vi "Switch Unflatten Test Parameters.vi"(9 "error in (no error)":errorcluster, 10 "Parameter String":string) -> (1 "error out":errorcluster, 2 "Switch Test Parameters":T2, 5 "Test Version":string)   [LabVIEW 2011]
uses:
  TypeDefs/Switch Test Parameters.ctl
  TypeDefs/Switch Stimulus Parameters.ctl
  TypeDefs/Switch Type.ctl
  TypeDefs/Switch Instrument Info.ctl
  Test Return Parameter.ctl
  TypeDefs/Switch Test Parameters v5.3-5.4.ctl
  TypeDefs/Switch Test Parameters v5.5.ctl
panel:
  in  "Return Parameter":T1
  out "Parameter Variant":variant
  in  "Required Instruments":string[](array[string])=["SWI_PFE"]
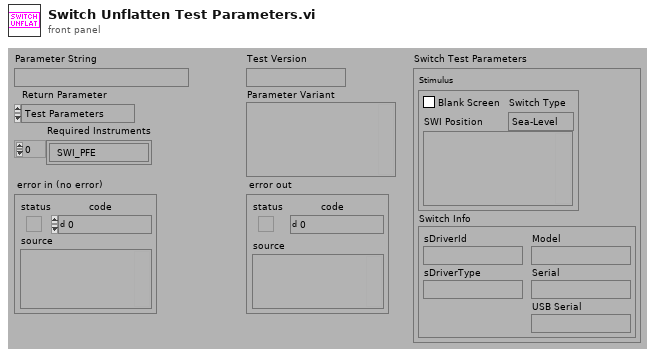
[diagram p1: front panel]
types:
  T1 = typedef "Test Return Parameter.ctl" = enum16{"Test Parameters", "Required Instruments", "Datasheets", "QuickMode"}
  T2 = typedef "Switch Test Parameters.ctl" = cluster{"Stimulus":T3, "Switch Info":T5}
  T3 = typedef "Switch Stimulus Parameters.ctl" = cluster{"Blank Screen":bool, "SWI Position":variant, "Switch Type":T4}
  T4 = typedef "Switch Type.ctl" = enum16{"Sea-Level", "Simulator", "SI-0206-SW", "SI-0309-SW", "SI-0310-SW", "Front End"}
  T5 = typedef "Switch Instrument Info.ctl" = cluster{"sDriverId":string, "sDriverType":string, "Model":string, "Serial":string, "USB Serial":string}
  T6 = typedef "Switch Test Parameters v5.3-5.4.ctl" = cluster{"Stimulus":cluster{"Blank Screen":bool, "SWI Position":variant}, "Switch Info":cluster{"sDriverId":string, "Model":string, "Serial":string}}
  T7 = typedef "Switch Test Parameters v5.5.ctl" = cluster{"Stimulus":cluster{"Blank Screen":bool, "SWI Position":variant, "Switch Type":enum16{"Sea-Level", "Simulator", "SI-0206-SW", "SI-0310-SW", "Front End"}}, "Switch Info":cluster{"sDriverId":string, "sDriverType":string, "Model":string, "Serial":string, "USB Serial":string}}
  T8 = enum16{"Sea-Level", "Simulator", "SI-0206-SW", "SI-0310-SW", "Front End"}
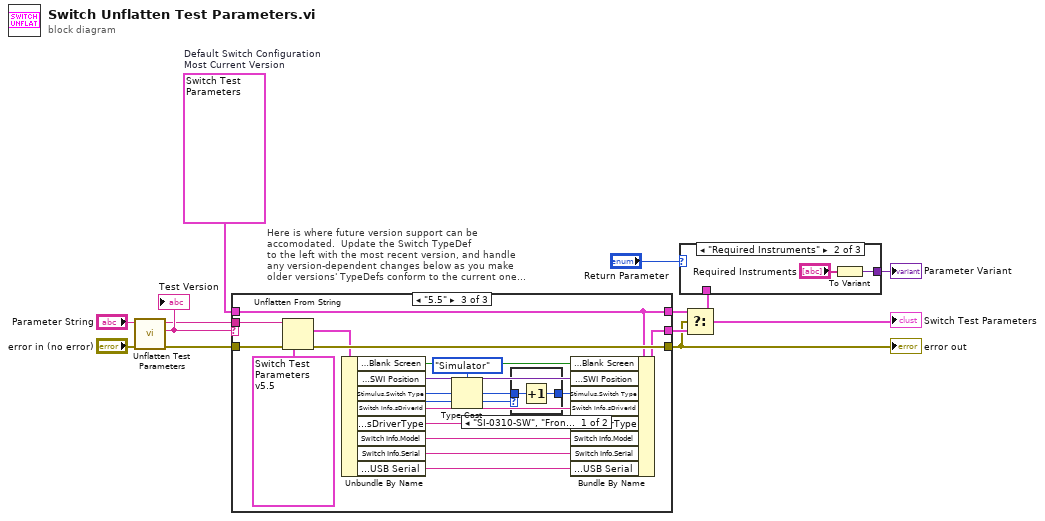
[diagram p0: block diagram]
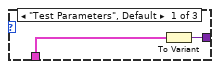
[diagram p2: hidden frame]
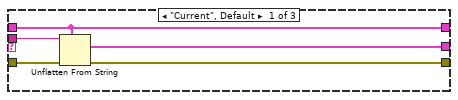
[diagram p4: hidden frame]
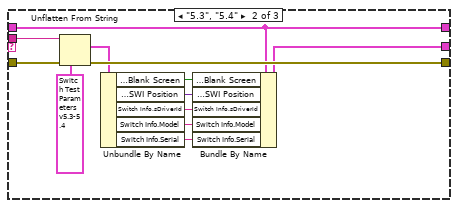
[diagram p5: hidden frame]
diagram:
  w2 = T2 {"Stimulus"={"Blank Screen"=FALSE, "SWI Position"=variant, "Switch Type"=enum."Simulator"}, "Switch Info"={"sDriverId"="", "sDriverType"="", "Model"="", "Serial"="", "USB Serial"=""}}  # Default Switch Configuration Most Current Version
  # "Here is where future version support can be\naccomodated.  Update the Switch TypeDef\nto the left with the most recent version, and handle\nany version-dependent changes below as you make\nolder versions' TypeDefs conform to the current one..."
  n1 = call "Unflatten Test Parameters.vi"("error in (no error)"="error in (no error)", "Flattened Test Parameters with Version (\"\")"="Parameter String") -> ("error out"=w3:errorcluster, "Test Version"=w11:string, "Flat Test Parameters"=w10:string)  [unwired: 3 out]
  "Test Version" <- w11
  n2 = case shown="\"5.5\"" w11 {
    tunnel: [w16 w23 w42] -> w9
    tunnel: w10 -> [w17 w29 w47]
    tunnel: [w14 w27 w45] -> w4
    tunnel: w3 -> [w15 w28 w46]
    tunnel: w2 -> [w13 w24 w43]
    tunnel: [w13 w24 w43] -> w1
    frame "Current", Default {
      n3 = Unflatten From String(type=w13, binary string=w17, error in (no error)=w15) -> (value=w16:T2, error out=w14:errorcluster)  [unwired: 3 out]
    }
    frame "5.3", "5.4" {
      n4 = Unflatten From String(type=T6 {"Stimulus"={"Blank Screen"=FALSE, "SWI Position"=variant}, "Switch Info"={"sDriverId"="", "Model"="", "Serial"=""}} ("Switch Test Parameters"), binary string=w29, error in (no error)=w28) -> (value=w25:T6, error out=w27:errorcluster)  [unwired: 3 out]
      n5 = Unbundle By Name(w25) -> ("Stimulus.Blank Screen"=w22:bool, "Stimulus.SWI Position"=w21:variant, "Switch Info.sDriverId"=w20:string, "Switch Info.Model"=w19:string, "Switch Info.Serial"=w18:string)
      n6 = Bundle By Name(cluster=w24, "Stimulus.Blank Screen"=w22, "Stimulus.SWI Position"=w21, "Switch Info.sDriverId"=w20, "Switch Info.Model"=w19, "Switch Info.Serial"=w18) -> (w23:T2)
    }
    frame "5.5" {
      n7 = Unflatten From String(type=T7 {"Stimulus"={"Blank Screen"=FALSE, "SWI Position"=variant, "Switch Type"=enum."Simulator"}, "Switch Info"={"sDriverId"="", "sDriverType"="", "Model"="", "Serial"="", "USB Serial"=""}} ("Switch Test Parameters"), binary string=w47, error in (no error)=w46) -> (value=w44:T7, error out=w45:errorcluster)  [unwired: 3 out]
      n8 = Unbundle By Name(w44) -> ("Stimulus.Blank Screen"=w41:bool, "Stimulus.SWI Position"=w40:variant, "Stimulus.Switch Type"=w32:T8, "Switch Info.sDriverId"=w38:string, "Switch Info.sDriverType"=w37:string, "Switch Info.Model"=w36:string, "Switch Info.Serial"=w35:string, "Switch Info.USB Serial"=w34:string)
      n9 = Type Cast(type=Switch_Type."Simulator" ("Stimulus.Switch Type"), x=w32) -> (*(type *) &x=w31:T4)
      n10 = case shown="\"SI-0310-SW\", \"Front End\"" w32 {
        tunnel: w31 -> [w49 w50]
        tunnel: [w48 w50] -> w30
        frame "SI-0310-SW", "Front End" {
          n11 = Increment(x=w49) -> (x+1=w48:T4)
        }
        frame Default {
        }
      }
      n12 = Bundle By Name(cluster=w43, "Stimulus.Blank Screen"=w41, "Stimulus.SWI Position"=w40, "Stimulus.Switch Type"=w30, "Switch Info.sDriverId"=w38, "Switch Info.sDriverType"=w37, "Switch Info.Model"=w36, "Switch Info.Serial"=w35, "Switch Info.USB Serial"=w34) -> (w42:T2)
    }
  }
  "error out" <- w4
  n13 = Select(t=w1, s=w4, f=w9) -> (s? t:f=w6:T2)
  "Switch Test Parameters" <- w6
  n14 = case shown="\"Required Instruments\"" "Return Parameter" {
    tunnel: [w52 w54 _] -> w7
    tunnel: w6 -> [w51 _ _]
    frame "Test Parameters", Default {
      n15 = To Variant(anything=w51) -> (Variant=w52:variant)
    }
    frame "Required Instruments" {
      n16 = To Variant(anything="Required Instruments") -> (Variant=w54:variant)
    }
    frame "Datasheets", "QuickMode" {
    }
  }
  "Parameter Variant" <- w7
